vi "_TangoWriteAttributes.vi"(1 "error in":errorcluster, 2 "attribute Values":T1(array[cluster]), 3 "device name":string) -> (0 "error out":errorcluster)   [LabVIEW 2014, in "tango.lvlib"]
uses:
  tango.lvlib
  tango_binding.so
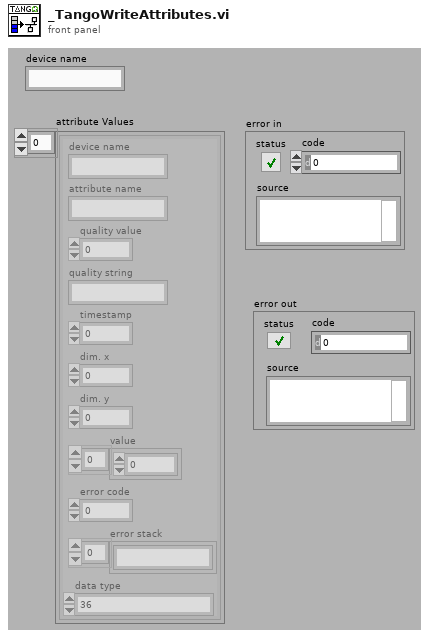
[diagram p1: front panel]
types:
  T1 = cluster{"device name":string, "attribute name":string, "quality value":i16, "quality string":string, "timestamp":dbl, "dim. x":i32, "dim. y":i32, "value":u8[], "error code":i32, "error stack":string[], "data type":u16}[]
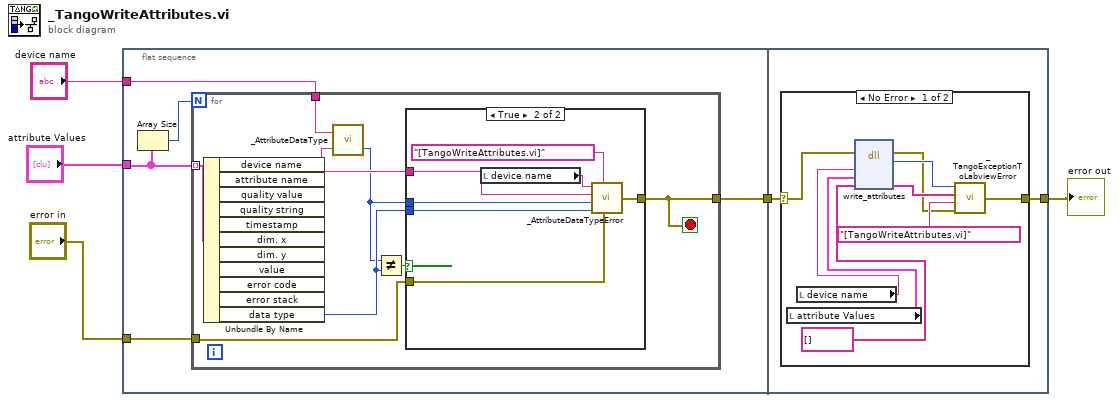
[diagram p0: block diagram]
diagram:
  n1 = flat-sequence {
    tunnel: "device name" -> [w10]
    tunnel: "attribute Values" -> [w8]
    tunnel: "error in" -> [w7]
    tunnel: [w6] -> w3
    tunnel: w3 -> [w28]
    tunnel: [w27] -> w2
    frame #0 {
      n2 = Array Size(array=w8) -> (size(s)=w9:i32)
      n3 = for {
        N: w9 -> [_]
        tunnel: w10 -> [w18]
        tunnel: w8 -> [w16] mode=indexing
        tunnel: w7 -> [w13]
        tunnel: [w12] -> w6
        stop <- w12 stop-if-true
        n4 = Unbundle By Name(w16) -> ("attribute name"=w15:string, "data type"=w14:u16)  [unwired: 9 out]
        n5 = call "_AttributeDataType.vi"("attribute name"=w15, "device name"=w18) -> ("data type value"=w11:u16)  [unwired: 1 out]
        n6 = Not Equal?(x=w11, y=w14) -> (x != y?=w17:bool)
        n7 = case shown="True" w17 {
          tunnel: w15 -> [_ w26]
          tunnel: w14 -> [_ w21]
          tunnel: w13 -> [w19 w23]
          tunnel: [w19 w24] -> w12
          tunnel: w11 -> [_ w20]
          frame False {
          }
          frame True {
            n8 = local read "device name"() -> (w25:string)
            n9 = call "_AttributeDataTypeError.vi"("error in"=w23, "location"="[TangoWriteAttributes.vi]", "user Data Type"=w21, "actual Data Type"=w20, "attribute name"=w26, "device name"=w25) -> ("error out"=w24:errorcluster)
          }
        }
      }
    }
    frame #1 {
      n10 = case shown="No Error" w28 {
        selector: w28 -> [w33 w38]
        tunnel: [w29 w38] -> w27
        frame No Error {
          n11 = local read "attribute Values"() -> (w31:T1)
          n12 = local read "device name"() -> (w32:string)
          n13 = dll-call lib="tango_binding.*" fn="write_attributes"(error in=w33, "device_name"=w32, "attr_values_inout"=w31, "error_stack"=string[] [] ("error stack")) -> (error out=w34:errorcluster, "type de retour"=w35:i32, "error_stack"=w36:string[])  [unwired: 4 in, 1 out]
          n14 = call "_TangoExceptionToLabviewError.vi"("error in"=w34, "location"="[TangoWriteAttributes.vi]", "error stack"=w36, "error code"=w35) -> ("error out"=w29:errorcluster)
        }
        frame Error {
        }
      }
    }
  }
  "error out" <- w2
